vi "cluster.vi"() -> ()   [LabVIEW 2025]
panel:
  out "workshop attended 2":bool
  out "Year of study":dbl
  out "Roll no":dbl
  out "Student Name":string
  in  "PACE":T1
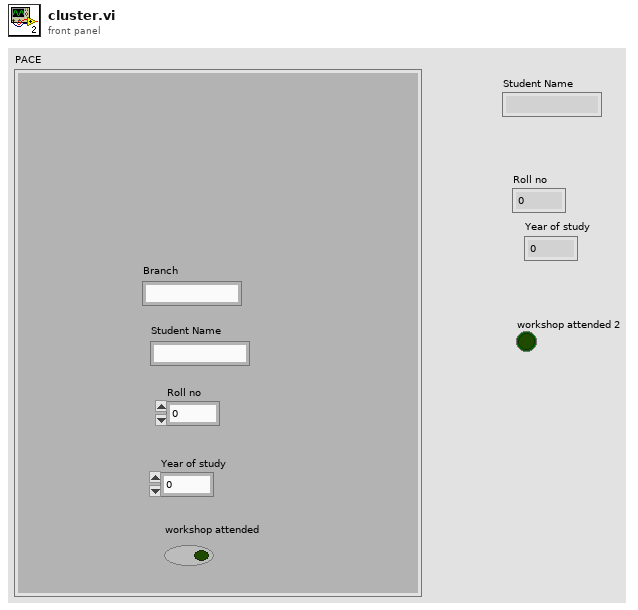
[diagram p1: front panel]
types:
  T1 = cluster{"Branch":string, "Student Name":string, "Roll no":dbl, "Year of study":dbl, "workshop attended":bool}
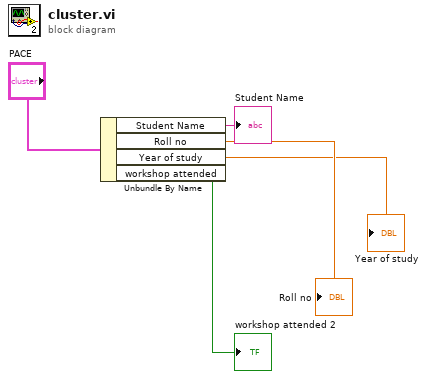
[diagram p0: block diagram]
diagram:
  n1 = Unbundle By Name "Unbundle By Name"("PACE") -> ("Student Name"=→"Student Name":string, "Roll no"=→"Roll no":dbl, "Year of study"=→"Year of study":dbl, "workshop attended"=→"workshop attended 2":bool)
